vi "CRYUpdate Curve from Jump.vi"(10 "Y Value":dbl, 11 "Step Configure":T2={"No.VI"=0, "Category"="", "StepName"="", "Seq setup flattened"="", "Comment"="", "Steps config."=[], "Jump config"=[], "Start"=0.0, "Increment"=0.0, "Name"="Pa", "Unit"="Pa", "Y data"=1, "Y prefix"="", "Y dB ref"=1.0, "Y unit"="", "Repeat State Array"=[]} {"Repeat State Array"."Start" format="%#_5g"; "Y dB ref" format="%.1f"; "Y data" items=["dB", "Lin"]; "Start" format="%#_5g"}) -> (3 "Inserted Names Out":string[](array[string]))   [LabVIEW 2013]
uses:
  CRYSystem/Typedef Control/CRYStep.ctl
  CRYSystem/Typedef Control/CRYData Cluster.ctl
panel:
  in  "Value":cluster{"x":dbl, "y":dbl, "z":dbl} {"z" format="%.2f"; "y" format="%.2f"; "x" format="%.2f"}
  in  "Datum":T1={"Name"="", "Curve"=[], "X data"=1, "Y data"=1, "Z data"=1, "X axis"=0, "Y axis"=1, "Z axis"=1, "X unit"="Hz", "Y unit"="", "Z unit"="deg.", "X dB ref"=1.0, "Y dB ref"=1.0, "Z dB ref"=1.0, "single val"=FALSE, "protected"=FALSE, "display X"=TRUE, "display Y"=TRUE, "display Z"=TRUE, "Test Info"="", "Step No."=0, "Plot Settings"={"Color"=0, "Interpolation"=0, "Point Style"=0, "Line Style"=0, "Point Color"=0, "Line Width"=0, "Bar Plot Style"=0, "Fill To"=0}, "AutoProtect"=FALSE} {"Z data" items=["dB", "Lin"]; "X data" items=["dB", "Lin"]; "Y data" items=["dB", "Lin"]; "Z dB ref" format="%.1f"; "Z axis" items=["Log", "Lin"]; "X dB ref" format="%.1f"; "X axis" items=["Log", "Lin"]; "Y axis" items=["Log", "Lin"]; "Y dB ref" format="%.1f"; "Curve"."z" format="%.2f"; "Curve"."y" format="%.2f"; "Curve"."x" format="%.2f"}
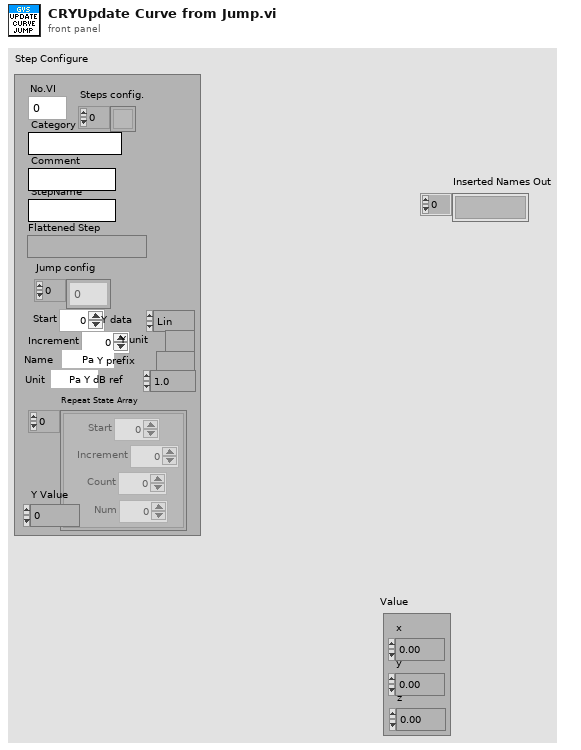
[diagram p1: front panel]
types:
  T1 = typedef "CRYData Cluster.ctl" = cluster{"Name":string, "Curve":cluster{"x":dbl, "y":dbl, "z":dbl}[], "X data":u16, "Y data":u16, "Z data":u16, "X axis":u16, "Y axis":u16, "Z axis":u16, "X unit":string, "Y unit":string, "Z unit":string, "X dB ref":dbl, "Y dB ref":dbl, "Z dB ref":dbl, "single val":bool, "protected":bool, "display X":bool, "display Y":bool, "display Z":bool, "Test Info":string, "Step No.":i32, "Plot Settings":cluster{"Color":u32, "Interpolation":u8, "Point Style":u8, "Line Style":u8, "Point Color":u32, "Line Width":u8, "Bar Plot Style":u8, "Fill To":i16}, "AutoProtect":bool}
  T2 = typedef "CRYStep.ctl" = cluster{"No.VI":i32, "Category":string, "StepName":string, "Seq setup flattened":string, "Comment":string, "Steps config.":bool[], "Jump config":i32[], "Start":dbl, "Increment":dbl, "Name":string, "Unit":string, "Y data":u16, "Y prefix":string, "Y dB ref":dbl, "Y unit":string, "Repeat State Array":cluster{"Start":dbl, "Increment":dbl, "Count":i32, "Num":i32}[]}
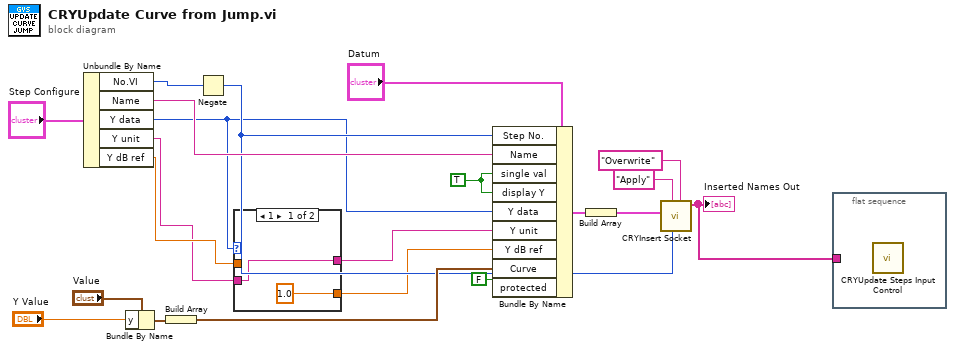
[diagram p0: block diagram]
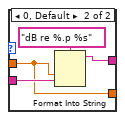
[diagram p2: hidden frame]
diagram:
  w18 = TRUE ("single val")
  n1 = Unbundle By Name("Step Configure") -> ("No.VI"=w13:i32, "Name"=w19:string, "Y data"=w9:u16, "Y unit"=w7:string, "Y dB ref"=w8:dbl)
  n2 = Bundle By Name(cluster="Value", "y"="Y Value") -> (w16:cluster{"x":dbl, "y":dbl, "z":dbl})
  n3 = Build Array(w16) -> (w15:cluster{"x":dbl, "y":dbl, "z":dbl}[])
  n4 = Negate(x=w13) -> (-x=w10:i32)
  n5 = case shown="1" w9 {
    tunnel: [w23 w25] -> w6
    tunnel: w8 -> [_ w24]
    tunnel: w7 -> [w23 w26]
    tunnel: [1.0 ("dB ref Out") w24] -> w5
    frame 1 {
    }
    frame 0, Default {
      n6 = Format Into String(format string="dB re %.p %s", w24, w26) -> (resulting string=w25:string)  [unwired: 2 in, 1 out]
    }
  }
  n7 = Bundle By Name(cluster="Datum", "Step No."=w10, "Name"=w19, "single val"=w18, "display Y"=w18, "Y data"=w9, "Y unit"=w6, "Y dB ref"=w5, "Curve"=w15, "protected"=FALSE) -> (w12:T1)
  n8 = Build Array(w12) -> (w11:T1[])
  n9 = call "CRYInsert Socket.vi"("sOption2"="Overwrite", "Step No."=w10, "sOption1"="Apply", "Values"=w11) -> ("Inserted Names Out"=w1:string[])  [unwired: 7 in]
  "Inserted Names Out" <- w1
  n10 = flat-sequence {
    tunnel: w1 -> [_]
    frame #0 {
      n11 = call "CRYUpdate Steps Input Control.vi"() -> ()  [unwired: 12 in]
    }
  }
